vi "ModbusTxLoop.vi"(11 "ModbusPortSettings":T1={"TxPort"="ModbusPort1Tx", "TxDataFIFO"="ModbusPort1TxFIFO", "TxInternalDataFIFO"="ModbusPort1TxInternalFIFO", "TxHealthAndStatusFIFO"="ModbusPort1TxHealthAndStatusFIFO", "RxPort"="ModbusPort1Rx", "RxDataFIFO"="ModbusPort1RxFIFO", "RxHealthAndStatusFIFO"="ModbusPort1RxHealthAndStatusFIFO", "WaitForRxFrameRegister"="ModbusPort1WaitForRxControl", "BaseHealthAndStatusAddress"=0, "IRQAddress"=0, "TriggerIRQRegister"="ModbusPort1IRQControl", "SoftwareControlledTrigger"="ModbusSoftwareControlledTrigger", "TimestampRegister"="TimestampRegister", "TxTimestampFIFO"="ModbusPort1TimestampFIFO"}) -> ()   [LabVIEW 2016, in "FPGAModbus.lvlib"]
uses:
  FPGAModbus.lvlib
  DataTypes/ModbusPortSettings.ctl
  DataTypes/ModbusTxLoopData.ctl
  DataTypes/ModbusTxStates.ctl
  <vilib>/Platform/TimedLoop/XDataNode/timing_clust.ctl
  <vilib>/Platform/TimedLoop/XDataNode/nitl_modes.ctl
  <vilib>/Platform/TimedLoop/XDataNode/wakeup.ctl
  Common_FPGA_HealthAndStatus/DataTypes/HealthAndStatusUpdateMode.ctl
  <vilib>/rvi/Emulation/niFpgaSctlEmulationGetInTimedLoop.vi
  <vilib>/rvi/Emulation/niFpgaEmulationReportErrorSimple.vi
  <vilib>/rvi/Emulation/niFpgaGetClockAttributes.vi
  <vilib>/rvi/Emulation/niFpgaCriticalErrorInLSC.vi
  <vilib>/rvi/DataTransferAndStorage/Container/Common/niFpgaContainerExecOnDevCompGetState.vi
  <vilib>/rvi/Emulation/niFpgaEmulationIsFPGAContextNoSignature.vi
  <vilib>/rvi/errors/niFpgaSetErrorForExecOnDevCompSimple.vi
  <vilib>/rvi/eio/common/nirviEmuReportErrorAndStop.vi
  <vilib>/rvi/DataTransferAndStorage/Container/Common/niFpgaContainerGetUniqueNameForEmu.vi
  <vilib>/rvi/FIFO/Fifo_Resource/nirvififoEmulationSetSize.vi
  <vilib>/rvi/FIFO/Fifo_Resource/nirviFifoEmulationQueueMgr.vi
  <instcachedir>/0/nirviFifoEmulationQueueMgr_E5CAEC123FF24DC58D834DCA3CDAA9B5.lvgen/nirviFifoEmulationQueueMgr_E5CAEC123FF24DC58D834DCA3CDAA9B5_010.vi
  <vilib>/rvi/FIFO/Fifo_Resource/nirvififoEmulationDetermineInputValidOut.vi
  <vilib>/rvi/FIFO/Fifo_Resource/nirvififoEmulationCreateLock.vi
  <vilib>/rvi/Emulation/niFpgaProcessEmulError.vi
  <vilib>/rvi/FIFO/Fifo_Resource/nirvififoEmulationObtainLock.vi
  <vilib>/rvi/FIFO/Fifo_Resource/nirvififoEmulationReleaseLock.vi
  <vilib>/rvi/occurrence/nirviWaitOnOccurrenceBase.vi
  <vilib>/rvi/errors/nirviReportUnexpectedCaseInternalError.vi
  <vilib>/rvi/errors/nirviReportUnexpectedCaseInternalError (U32).vi
  <vilib>/Utility/error.llb/Clear Errors.vi
  <vilib>/rvi/interface/RandomDataEmulation/niFpgaRandomDataHandleErrors.vi
  <vilib>/rvi/Memory/Memory_Emulation/niFpgaMemoryEmulationCacheClearOnFirstRun.vi
  <vilib>/rvi/Memory/Memory_Emulation/nirvimemoryEmulationManagerCache_MakeExclusive.vi
  <vilib>/rvi/Memory/Memory_Emulation/niFpgaMemoryEmulationValidateCache.vi
  <vilib>/rvi/Memory/Memory_Emulation/nirvimemoryEmulationManagerCache_InsertValue.vi
  <vilib>/rvi/Memory/Memory_Emulation/nirvimemoryEmulationManagerCache_ReleaseExclusive.vi
  <vilib>/rvi/Memory/Memory_Emulation/nirvimemoryEmulationManagerCache_GetValue.vi
  <vilib>/rvi/Memory/Memory_Emulation/nirvimemoryEmulationManagerCache_SetValue.vi
  <instcachedir>/0/nirviFifoEmulationQueueMgr_E5CAEC123FF24DC58D834DCA3CDAA9B5.lvgen/nirviFifoEmulationQueueMgr_E5CAEC123FF24DC58D834DCA3CDAA9B5_007.vi
  <vilib>/rvi/eio/common/nirviEmuTemplateMethod_errors.vi
  <vilib>/Platform/TimedLoop/XDataNode/XDataNode.xnode
  <vilib>/rvi/DataTransferAndStorage/Container/XNode/niFpgaContainer.xnode
  <vilib>/rvi/FIFO/Fifo_Resource/niFpgaFifoEmulationRefIn.vi
  <vilib>/rvi/DataTransferAndStorage/Register/Emulation/niFpgaRegisterEmulationRefIn.vi
  <vilib>/eio/EIONode/EIONode.xnode
  Common_FPGA_HealthAndStatus/FPGAHealthAndStatus.lvlib
  <vilib>/Platform/TimedLoop/XDataNode/XDNodeRunTimeDep.lvlib
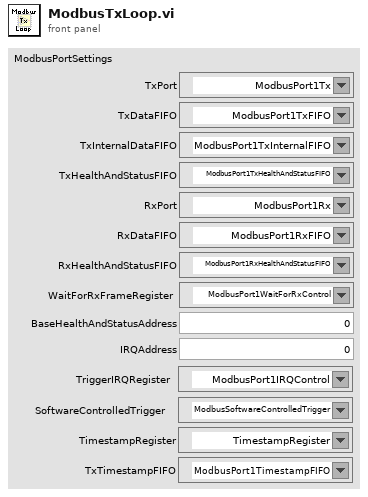
[diagram p1: front panel]
types:
  T1 = typedef "FPGAModbus.lvlib/ModbusPortSettings.ctl" = cluster{"TxPort":refnum<k21>, "TxDataFIFO":refnum<k21>, "TxInternalDataFIFO":refnum<k21>, "TxHealthAndStatusFIFO":refnum<k21>, "RxPort":refnum<k21>, "RxDataFIFO":refnum<k21>, "RxHealthAndStatusFIFO":refnum<k21>, "WaitForRxFrameRegister":refnum<k21>, "BaseHealthAndStatusAddress":u32, "IRQAddress":u8, "TriggerIRQRegister":refnum<k21>, "SoftwareControlledTrigger":refnum<k21>, "TimestampRegister":refnum<k21>, "TxTimestampFIFO":refnum<k21>}
  T2 = typedef "FPGAModbus.lvlib/ModbusTxLoopData.ctl" = cluster{"State":T3, "WriteData":u16, "DelayTicks":u32, "StateAfterDelay":T3, "Bit":u16, "BytesSent":u16}
  T3 = typedef "FPGAModbus.lvlib/ModbusTxStates.ctl" = enum16{"TryReadInstruction", "Delay", "WriteBits", "WaitForRxFrame", "WaitForTrigger", "ClearIRQFlag"}
  T4 = typedef "XDNodeRunTimeDep.lvlib/timing_clust.ctl" = cluster{"Expected End [f-1]":u64, "Actual End [f-1]":u64, "Finished Late? [f-1]":bool, "Expected End [i-1]":u64, "Actual End [i-1]":u64, "Finished Late? [i-1]":bool, "Expected Start [i]":u64, "Actual Start [i]":u64, "Expected Start [f]":u64, "Actual Start [f]":u64, "Source Name":string, "Structure Name":string, "Period":i64, "Deadline":i64, "Offset":i64, "Start":i64, "Priority":i32, "Timeout":i32, "Mode":T5, "Wakeup Reason":T6, "Error":errorcluster, "Source Type":string, "Secondary Source Type":string, "Global End Time":u64, "Global Start Time":u64, "Frame Duration":u64, "Iteration Duration":u64, "Assigned CPU":i32, "I/O Scan Engine Mode":u32}
  T5 = typedef "XDNodeRunTimeDep.lvlib/nitl_modes.ctl" = enum32{"No Change", "Process missed periods, maintain original phase", "Discard missed periods, maintain original phase", "Process missed periods, ignore original phase", "Discard missed periods, ignore original phase"}
  T6 = typedef "XDNodeRunTimeDep.lvlib/wakeup.ctl" = enum32{"Normal", "Aborted", "Asynchronous wakeup", "Timing source error", "Timed loop error", "Timeout"}
  T7 = typedef "FPGAHealthAndStatus.lvlib/HealthAndStatusUpdateMode.ctl" = enum8{"NOP", "Set", "Add", "Subtract", "Or"}
  T8 = cluster{"InstructionType":enum8{"NOP", "WriteByte", "EndOfFrame", "PushTimestamp", "DelayMicroseconds", "DelayMilliseconds", "WaitForRxFrame", "TriggerIRQ", "WaitForTrigger", "WaitForLongRxFrame"}, "Data":u16}
  T9 = enum8{"NOP", "WriteByte", "EndOfFrame", "PushTimestamp", "DelayMicroseconds", "DelayMilliseconds", "WaitForRxFrame", "TriggerIRQ", "WaitForTrigger", "WaitForLongRxFrame"}
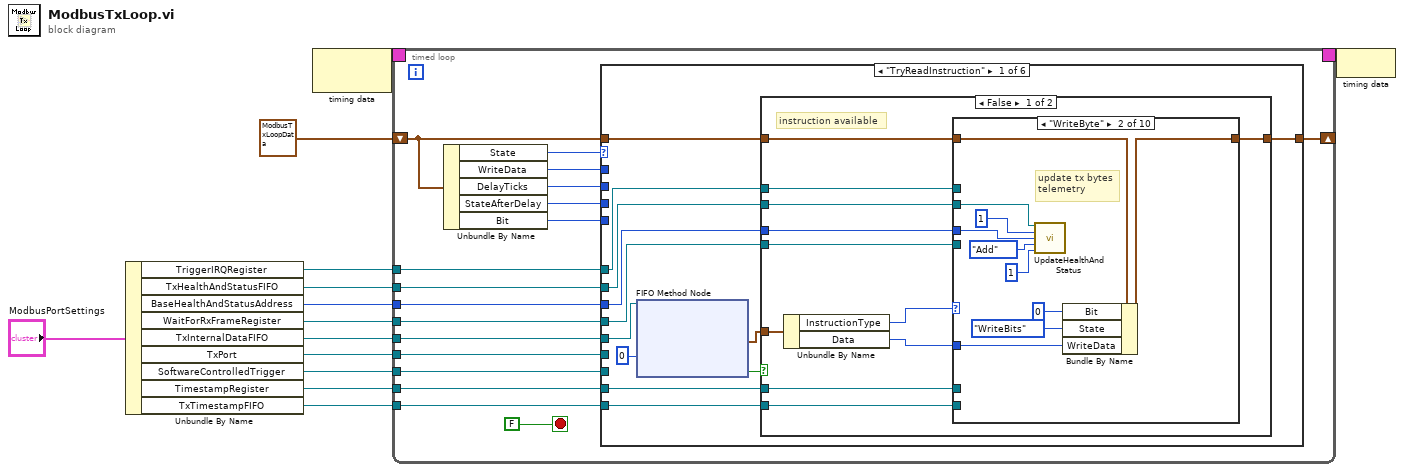
[diagram p0: block diagram]
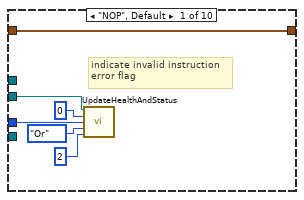
[diagram p2: hidden frame]
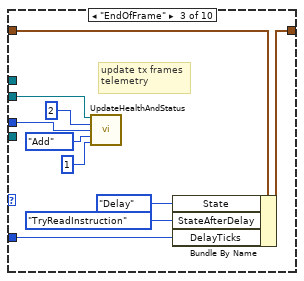
[diagram p3: hidden frame]
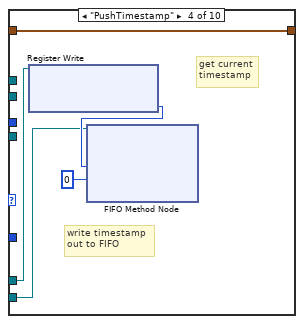
[diagram p4: hidden frame]
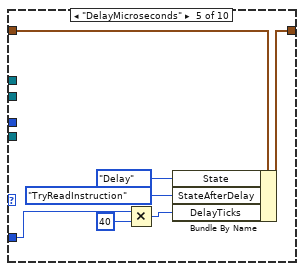
[diagram p5: hidden frame]
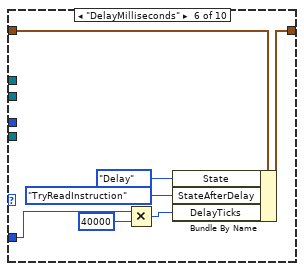
[diagram p6: hidden frame]
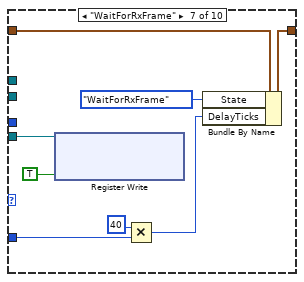
[diagram p7: hidden frame]
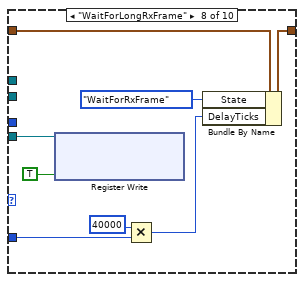
[diagram p8: hidden frame]
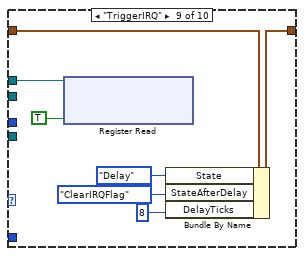
[diagram p9: hidden frame]
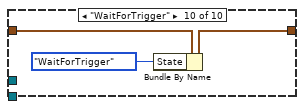
[diagram p10: hidden frame]
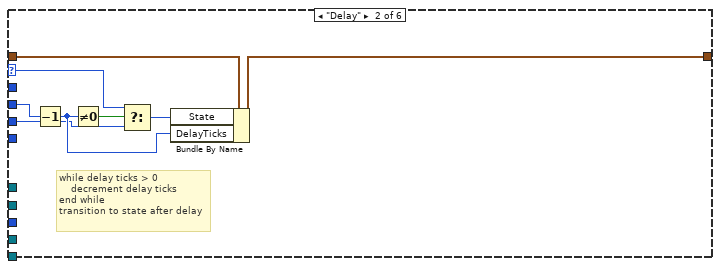
[diagram p12: hidden frame]
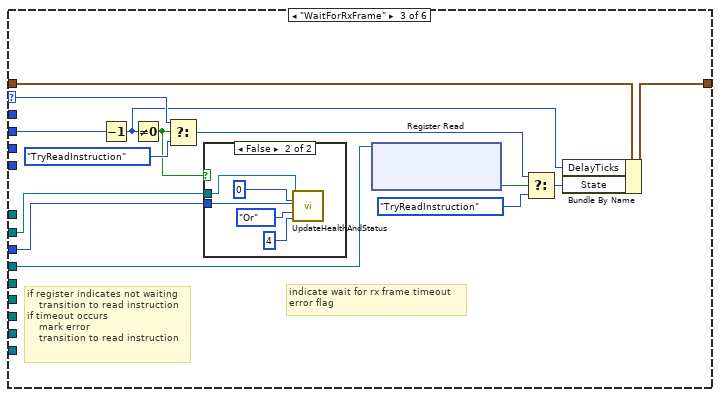
[diagram p13: hidden frame]
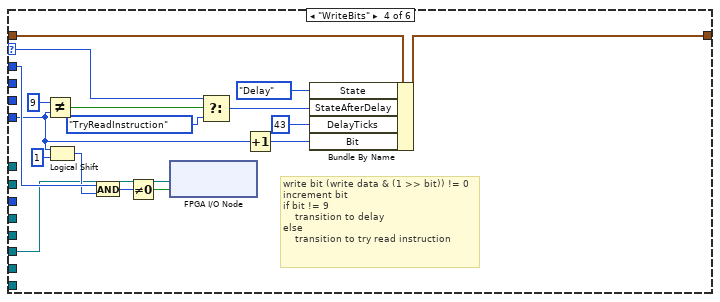
[diagram p15: hidden frame]
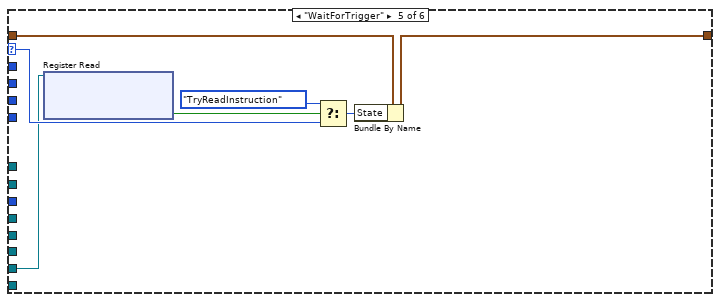
[diagram p16: hidden frame]
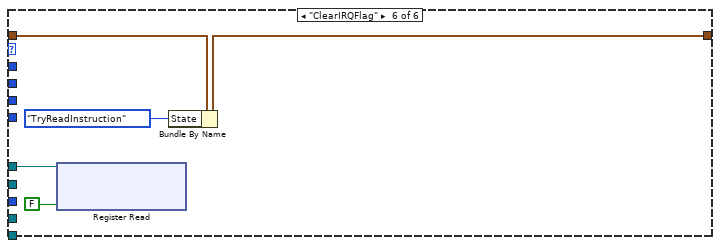
[diagram p17: hidden frame]
diagram:
  n1 = Unbundle By Name("ModbusPortSettings") -> ("TriggerIRQRegister"=w11:refnum<k21>, "TxHealthAndStatusFIFO"=w6:refnum<k21>, "BaseHealthAndStatusAddress"=w7:u32, "WaitForRxFrameRegister"=w8:refnum<k21>, "TxInternalDataFIFO"=w9:refnum<k21>, "TxPort"=w10:refnum<k21>, "SoftwareControlledTrigger"=w3:refnum<k21>, "TimestampRegister"=w2:refnum<k21>, "TxTimestampFIFO"=w1:refnum<k21>)
  n2 = node-c288() -> (w13:T4)  [unwired: 1 in]
  n3 = timed-loop {
    shift-right: [w30] -> _
    shift-left: T2 {"State"=enum."TryReadInstruction", "WriteData"=0, "DelayTicks"=0, "StateAfterDelay"=enum."TryReadInstruction", "Bit"=0, "BytesSent"=0} ("ModbusTxLoop") -> [w29]
    tunnel: w8 -> [w27]
    tunnel: w7 -> [w23]
    tunnel: w6 -> [w21]
    timing: w13 -> [_]
    timing-out: [_] -> w12
    tunnel: w9 -> [w20]
    tunnel: w10 -> [w19]
    tunnel: w11 -> [w18]
    tunnel: w3 -> [w16]
    tunnel: w2 -> [w15]
    tunnel: w1 -> [w14]
    stop <- FALSE stop-if-true
    n4 = Unbundle By Name(w29) -> ("State"=w28:T3, "WriteData"=w26:u16, "DelayTicks"=w25:u32, "StateAfterDelay"=w24:T3, "Bit"=w22:u16)
    n5 = case shown="\"TryReadInstruction\"" w28 {
      selector: w28 -> [_ w129 w140 w163 w172 _]
      tunnel: w29 -> [w42 w133 w145 w166 w175 w179]
      tunnel: [w41 w132 w144 w161 w174 w178] -> w30
      tunnel: w27 -> [w40 _ w142 _ _ _]
      tunnel: w26 -> [_ _ _ w168 _ _]
      tunnel: w25 -> [_ w131 w141 _ _ _]
      tunnel: w24 -> [_ w126 _ _ _ _]
      tunnel: w23 -> [w39 _ w134 _ _ _]
      tunnel: w22 -> [_ _ _ w156 _ _]
      tunnel: w21 -> [w38 _ w135 _ _ _]
      tunnel: w20 -> [w36 _ _ _ _ _]
      tunnel: w19 -> [_ _ _ w153 _ _]
      tunnel: w18 -> [w37 _ _ _ _ w181]
      tunnel: w16 -> [_ _ _ _ w170 _]
      tunnel: w15 -> [w32 _ _ _ _ _]
      tunnel: w14 -> [w31 _ _ _ _ _]
      frame "TryReadInstruction" {
        n6 = xnode ("FIFO Method Node")("Timeout"=0, "FIFO In"=w36) -> ("Element"=w33:T8, "Timed Out?"=w34:bool)  [unwired: 1 out]
        n7 = case shown="False" w34 {
          tunnel: w33 -> [w45 _]
          tunnel: w42 -> [w53 w125]
          tunnel: [w52 w125] -> w41
          tunnel: w39 -> [w51 _]
          tunnel: w38 -> [w50 _]
          tunnel: w40 -> [w47 _]
          tunnel: w37 -> [w46 _]
          tunnel: w32 -> [w44 _]
          tunnel: w31 -> [w43 _]
          frame False {
            # "instruction available"
            # "instruction available"
            n8 = Unbundle By Name(w45) -> ("InstructionType"=w48:T9, "Data"=w49:u16)
            n9 = case shown="\"WriteByte\"" w48 {
              tunnel: w49 -> [_ w68 w78 _ w87 w94 w101 w109 _ _]
              tunnel: w53 -> [w59 w69 w79 w84 w91 w98 w106 w114 w116 w124]
              tunnel: [w59 w67 w76 w84 w89 w96 w105 w113 w115 w122] -> w52
              tunnel: w51 -> [w55 w61 w71 _ _ _ _ _ _ _]
              tunnel: w50 -> [w54 w60 w70 _ _ _ _ _ _ _]
              tunnel: w47 -> [_ _ _ _ _ _ w102 w110 _ _]
              tunnel: w46 -> [_ _ _ _ _ _ _ _ w121 _]
              tunnel: w44 -> [_ _ _ w81 _ _ _ _ _ _]
              tunnel: w43 -> [_ _ _ w80 _ _ _ _ _ _]
              frame "NOP", Default {
                # "indicate invalid instruction\nerror flag"
                # "nop"
                n10 = call "UpdateHealthAndStatus.vi"("InternalHealthAndStatusFIFO"=w54, "AddressOffset"=u32 0 ("x"), "BaseAddress"=w55, "HealthAndStatusUpdateMode"=HealthAndStatusUpdateMode."Or" ("Telemetry Update Mode"), "Data"=u64 2) -> ()  [unwired: 11 in]
              }
              frame "WriteByte" {
                # "update tx bytes\ntelemetry"
                # "transition to write bits"
                n11 = call "UpdateHealthAndStatus.vi"("InternalHealthAndStatusFIFO"=w60, "AddressOffset"=u32 1 ("x"), "BaseAddress"=w61, "HealthAndStatusUpdateMode"=HealthAndStatusUpdateMode."Add" ("Telemetry Update Mode"), "Data"=u64 1) -> ()  [unwired: 11 in]
                n12 = Bundle By Name(cluster=w69, "Bit"=u16 0, "State"=ModbusTxStates."WriteBits", "WriteData"=w68) -> (w67:T2)
              }
              frame "EndOfFrame" {
                # "update tx frames\ntelemetry"
                # "transition to delay"
                n13 = call "UpdateHealthAndStatus.vi"("InternalHealthAndStatusFIFO"=w70, "AddressOffset"=u32 2 ("x"), "BaseAddress"=w71, "HealthAndStatusUpdateMode"=HealthAndStatusUpdateMode."Add" ("Telemetry Update Mode"), "Data"=u64 1) -> ()  [unwired: 11 in]
                n14 = Bundle By Name(cluster=w79, "State"=ModbusTxStates."Delay" ("TransmitStates"), "StateAfterDelay"=ModbusTxStates."TryReadInstruction" ("TransmitStates"), "DelayTicks"=w78) -> (w76:T2)
              }
              frame "PushTimestamp" {
                # "get current\ntimestamp"
                # "write timestamp\nout to FIFO"
                # "transition to delay"
                n15 = xnode "Register Write"("Register In"=w81) -> ("Data"=w83:u64)  [unwired: 1 out]
                n16 = xnode ("FIFO Method Node")("Element"=w83, "Timeout"=0, "FIFO In"=w80) -> ()  [unwired: 2 out]
              }
              frame "DelayMicroseconds" {
                # "transition to delay"
                n17 = Multiply(x=w87, y=u32 40) -> (x*y=w85:u32)
                n18 = Bundle By Name(cluster=w91, "State"=ModbusTxStates."Delay" ("TransmitStates"), "StateAfterDelay"=ModbusTxStates."TryReadInstruction" ("TransmitStates"), "DelayTicks"=w85) -> (w89:T2)
              }
              frame "DelayMilliseconds" {
                # "transition to delay"
                n19 = Multiply(x=w94, y=u32 40000) -> (x*y=w92:u32)
                n20 = Bundle By Name(cluster=w98, "State"=ModbusTxStates."Delay" ("TransmitStates"), "StateAfterDelay"=ModbusTxStates."TryReadInstruction" ("TransmitStates"), "DelayTicks"=w92) -> (w96:T2)
              }
              frame "WaitForRxFrame" {
                # "transition to delay"
                n21 = xnode ("Register Write")("Data"=TRUE, "Register In"=w102) -> ()  [unwired: 1 out]
                n22 = Multiply(x=u32 40, y=w101) -> (x*y=w100:u32)
                n23 = Bundle By Name(cluster=w106, "State"=ModbusTxStates."WaitForRxFrame" ("TransmitStates"), "DelayTicks"=w100) -> (w105:T2)
              }
              frame "WaitForLongRxFrame" {
                # "transition to delay"
                n24 = xnode ("Register Write")("Data"=TRUE, "Register In"=w110) -> ()  [unwired: 1 out]
                n25 = Multiply(x=u32 40000, y=w109) -> (x*y=w108:u32)
                n26 = Bundle By Name(cluster=w114, "State"=ModbusTxStates."WaitForRxFrame" ("TransmitStates"), "DelayTicks"=w108) -> (w113:T2)
              }
              frame "TriggerIRQ" {
                # "transition to delay"
                n27 = xnode ("Register Read")("Data"=TRUE, "Register In"=w121) -> ()  [unwired: 1 out]
                n28 = Bundle By Name(cluster=w116, "State"=ModbusTxStates."Delay", "StateAfterDelay"=ModbusTxStates."ClearIRQFlag", "DelayTicks"=u32 8) -> (w115:T2)
              }
              frame "WaitForTrigger" {
                n29 = Bundle By Name(cluster=w124, "State"=ModbusTxStates."WaitForTrigger") -> (w122:T2)
              }
            }
          }
          frame True {
            # "no instruction available"
            # "no instruction available"
          }
        }
      }
      frame "Delay" {
        # "while delay ticks > 0\n    decrement delay ticks\nend while\ntransition to state after delay"
        n30 = Decrement(x=w131) -> (x-1=w127:u32)
        n31 = Not Equal To 0?(x=w127) -> (x != 0?=w130:bool)
        n32 = Select(t=w129, s=w130, f=w126) -> (s? t:f=w128:T3)
        n33 = Bundle By Name(cluster=w133, "State"=w128, "DelayTicks"=w127) -> (w132:T2)
      }
      frame "WaitForRxFrame" {
        # "indicate wait for rx frame timeout\nerror flag"
        # "if register indicates not waiting\n    transition to read instruction\nif timeout occurs\n    mark error\n    transition to read instruction"
        n34 = Decrement(x=w141) -> (x-1=w137:u32)
        n35 = Not Equal To 0?(x=w137) -> (x != 0?=w136:bool)
        n36 = Select(t=w140, s=w136, f=ModbusTxStates."TryReadInstruction") -> (s? t:f=w139:T3)
        n37 = case shown="False" w136 {
          tunnel: w135 -> [_ w151]
          tunnel: w134 -> [_ w150]
          frame True {
          }
          frame False {
            n38 = call "UpdateHealthAndStatus.vi"("InternalHealthAndStatusFIFO"=w151, "AddressOffset"=u32 0 ("x"), "BaseAddress"=w150, "HealthAndStatusUpdateMode"=HealthAndStatusUpdateMode."Or" ("Telemetry Update Mode"), "Data"=u64 4) -> ()  [unwired: 11 in]
          }
        }
        n39 = xnode ("Register Read")("Register In"=w142) -> ("Data"=w147:bool)  [unwired: 1 out]
        n40 = Select(t=w139, s=w147, f=ModbusTxStates."TryReadInstruction") -> (s? t:f=w143:T3)
        n41 = Bundle By Name(cluster=w145, "DelayTicks"=w137, "State"=w143) -> (w144:T2)
      }
      frame "WriteBits" {
        # "write bit (write data & (1 >> bit)) != 0\nincrement bit\nif bit != 9\n    transition to delay\nelse\n    transition to try read instruction"
        n42 = Not Equal?(x=u16 9, y=w156) -> (x != y?=w155:bool)
        n43 = Logical Shift(y=w156, x=u16 1) -> (x << y=w158:u16)
        n44 = And(x=w168, y=w158) -> (x .and. y?=w169:u16)
        n45 = Not Equal To 0?(x=w169) -> (x != 0?=w167:bool)
        n46 = xnode "FPGA I/O Node"("I/O Item"=w167, "FPGA I/O In"=w153) -> ()  [unwired: 1 out]
        n47 = Select(t=w163, s=w155, f=ModbusTxStates."TryReadInstruction" ("TransmitStates")) -> (s? t:f=w165:T3)
        n48 = Increment(x=w156) -> (x+1=w160:u16)
        n49 = Bundle By Name(cluster=w166, "State"=ModbusTxStates."Delay" ("TransmitStates"), "StateAfterDelay"=w165, "DelayTicks"=u16 43 ("Delay Ticks"), "Bit"=w160) -> (w161:T2)
      }
      frame "WaitForTrigger" {
        n50 = xnode ("Register Read")("Register In"=w170) -> ("Data"=w176:bool)  [unwired: 1 out]
        n51 = Select(t=ModbusTxStates."TryReadInstruction", s=w176, f=w172) -> (s? t:f=w173:T3)
        n52 = Bundle By Name(cluster=w175, "State"=w173) -> (w174:T2)
      }
      frame "ClearIRQFlag" {
        n53 = xnode ("Register Read")("Data"=FALSE, "Register In"=w181) -> ()  [unwired: 1 out]
        n54 = Bundle By Name(cluster=w179, "State"=ModbusTxStates."TryReadInstruction") -> (w178:T2)
      }
    }
  }
  n55 = node-c288(w12) -> ()
